vi "Indicators.vi"() -> ()   [LabVIEW 2018]
panel:
  in  "LimeLight_Pipeline":dbl
  in  "LimeLight_Cam_Mode":dbl
  in  "LimeLight_LED_Mode":dbl
  in  "Elevator_Goal_(in)":dbl
  out "Elevator_Motor_Failure":bool
  out "Check_Limit_Switch":bool
  out "End_Of_Match":bool
  out "Elevator_Moving":bool
  out "Compressor_State":bool
  out "State_Conflict":bool
  out "State_Conflict_Light":bool
  out "COM_Warning":bool
  out "Tilt_Interlock_Engaged":bool
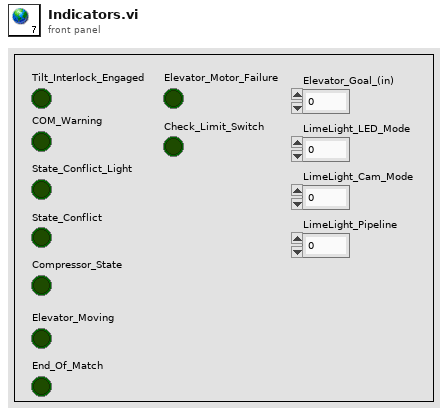
[diagram p1: front panel]
diagram:
